vi "Uv3_2022.vi"(1 "Gamma0 humid air":dbl, 2 "xw water mol fraction":dbl, 3 "Temperature [K]":dbl) -> (0 "Uv3":dbl)   [LabVIEW 2016]
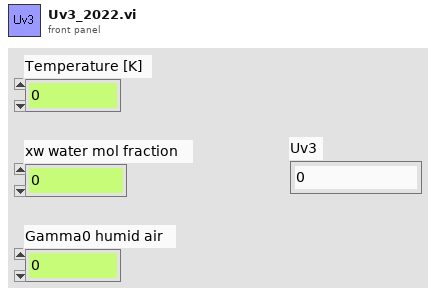
[diagram p1: front panel]
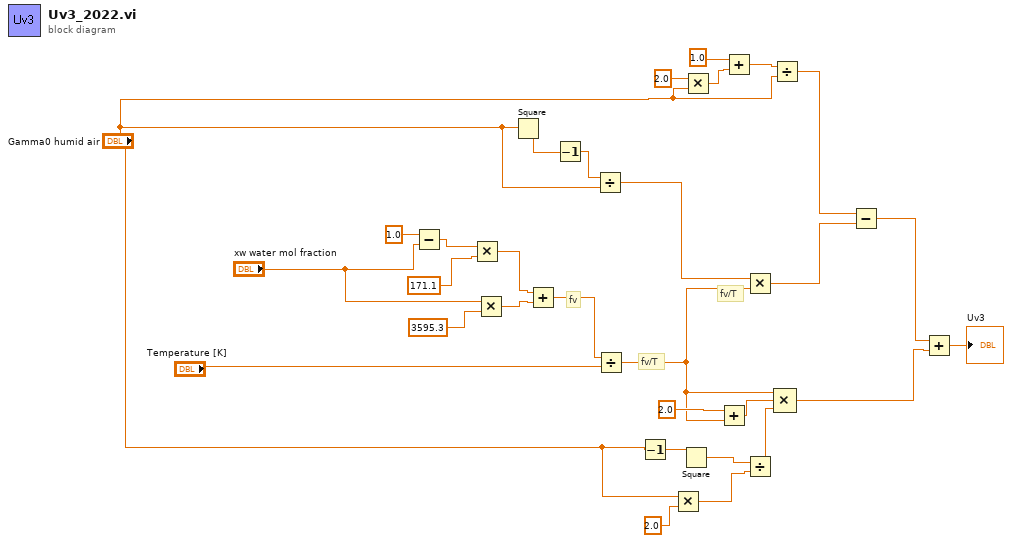
[diagram p0: block diagram]
diagram:
  # "fv/T"
  # "fv/T"
  # "fv"
  n1 = Subtract(x=1.0, y="xw water mol fraction") -> (x-y=w25:dbl)
  n2 = Multiply(x=w25, y=171.1) -> (x*y=w21:dbl)
  n3 = Multiply(x="xw water mol fraction", y=3595.3) -> (x*y=w20:dbl)
  n4 = Square(x="Gamma0 humid air") -> (x^2=w4:dbl)
  n5 = Add(x=w21, y=w20) -> (x+y=w19:dbl)
  n6 = Decrement(x=w4) -> (x-1=w3:dbl)
  n7 = Divide(x=w3, y="Gamma0 humid air") -> (x/y=w17:dbl)
  n8 = Divide(x=w19, y="Temperature [K]") -> (x/y=w12:dbl)
  n9 = Decrement(x="Gamma0 humid air") -> (x-1=w1:dbl)
  n10 = Multiply(x="Gamma0 humid air", y=2.0) -> (x*y=w8:dbl)
  n11 = Square(x=w1) -> (x^2=w10:dbl)
  n12 = Multiply(x=2.0, y="Gamma0 humid air") -> (x*y=w28:dbl)
  n13 = Add(x=2.0, y=w12) -> (x+y=w11:dbl)
  n14 = Add(x=1.0, y=w28) -> (x+y=w27:dbl)
  n15 = Multiply(x=w17, y=w12) -> (x*y=w15:dbl)
  n16 = Divide(x=w10, y=w8) -> (x/y=w7:dbl)
  n17 = Divide(x=w27, y="Gamma0 humid air") -> (x/y=w16:dbl)
  n18 = Compound Arithmetic op=MULTIPLY(w12, w11, w7) -> (w6:dbl)
  n19 = Subtract(x=w16, y=w15) -> (x-y=w14:dbl)
  n20 = Add(x=w14, y=w6) -> (x+y=→"Uv3":dbl)
